vi "ACT_LabVIEW1_Task2B_Team205.vi"() -> ()   [LabVIEW 2016]
uses:
  <vilib>/express/express arith-compare/Formula/XNode/ExpressFormulaBlockNode.xnode
panel:
  out "Numeric":dbl
  in  "p(inches)":dbl
  in  "u(inches)":dbl
  in  "L(inches)":dbl
  in  "V(inches)":dbl
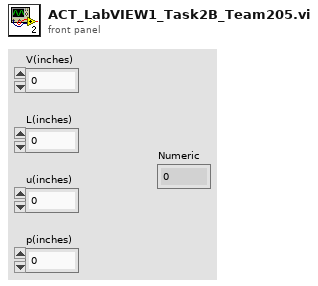
[diagram p1: front panel]
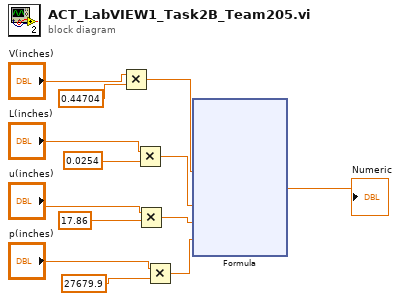
[diagram p0: block diagram]
diagram:
  n1 = Multiply(x="V(inches)", y=0.44704) -> (x*y=w4:dbl)
  n2 = Multiply(x="L(inches)", y=0.0254) -> (x*y=w3:dbl)
  n3 = Multiply(x="u(inches)", y=17.86) -> (x*y=w2:dbl)
  n4 = Multiply(x="p(inches)", y=27679.9) -> (x*y=w1:dbl)
  n5 = xnode "Formula"("V"=w4, "L"=w3, "u"=w2, "p"=w1) -> ("Result"=→"Numeric":dbl)  [unwired: 1 in, 1 out]
